vi "Master_NavigationLoop.vi"(8 "error in (no error)":errorcluster) -> (0 "error out":errorcluster)   [LabVIEW 2017]
uses:
  TypeDef_LoopPeriods.ctl
  DAQ/Master_DataControl.ctl
  DAQ/TypeDef_cRIOData.ctl
  IMU/TypeDef_IMUData.ctl
  CAN/TypeDef_BMSData.ctl
  CAN/TypeDef_BMS_Status.ctl
  CAN/MotorController/fixedMotorData.ctl
  CAN/MotorController/MotorStatus.ctl
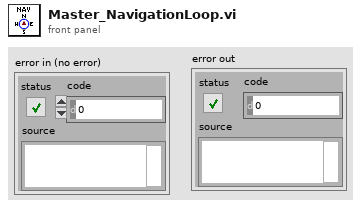
[diagram p1: front panel]
types:
  T1 = typedef "TypeDef_LoopPeriods.ctl" = cluster{"Control Period":i64, "DAQ Period":u32, "IMU Period":u32, "CAN Period":i64, "Nav Period":u32}
  T2 = typedef "Master_DataControl.ctl" = cluster{"cRIO Data":T3, "IMU Data":T4, "BMS Data":T5, "Motor Data":T7}
  T3 = typedef "TypeDef_cRIOData.ctl" = cluster{"Time (ms)":dbl, "24V Battery (V)":dbl, "LowV Current (A)":dbl, "Fiducial Sensor (V)":dbl, "PV Pressure (psig)":dbl, "Flow Sensor (V)":dbl, "Temp Fairing (F)":dbl, "Temp Reservoir (F)":dbl, "HallEffect Right (in)":dbl, "HallEffect Left (in)":dbl, "PT Tank (psig)":dbl, "PT Clamp Right (psig)":dbl, "PT Clamp Left (psig)":dbl, "PT Brake (psig)":dbl, "PT Cooling (psig)":dbl, "Displacement (ft)":dbl, "Velocity (ft/s)":dbl}
  T4 = typedef "TypeDef_IMUData.ctl" = cluster{"x acceleration (g)":dbl, "Pressure (psia)":dbl, "Temperature (F)":dbl}
  T5 = typedef "TypeDef_BMSData.ctl" = cluster{"Max Cell Voltage (V)":dbl, "Max Cell ID":dbl, "Min Cell Voltage (V)":dbl, "Min Cell ID":dbl, "State of Charge (%)":dbl, "Average Voltage (V)":dbl, "Voltage Delta (V)":dbl, "Pack Current (A)":dbl, "Pack Voltage (V)":dbl, "Max Resistance (Ohm)":dbl, "Min Resistance (Ohm)":dbl, "Average Resistance (Ohm)":dbl, "Delta Resistance (Ohm)":dbl, "Highest Temperature(F)":dbl, "BmsStatus":T6}
  T6 = typedef "TypeDef_BMS_Status.ctl" = cluster{"isFault":bool, "isolationMonitoring":bool}
  T7 = typedef "fixedMotorData.ctl" = cluster{"Velo (RPM)":dbl, "MotorTemp(F)":dbl, "CtrlTemp(F)":dbl, "DcLinkVolt(V)":dbl, "ErrorCode":dbl, "motorStatus":T8, "isAlive":bool, "motorControllerState":u16}
  T8 = typedef "MotorStatus.ctl" = cluster{"isReady":bool, "isOn":bool, "isOperEn":bool, "isFault":bool, "isVoltEn":bool, "targetReached":bool, "isWarning":bool}
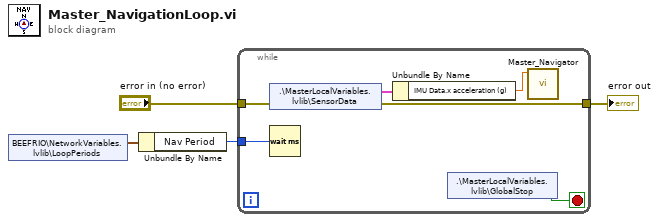
[diagram p0: block diagram]
diagram:
  n1 = shared-variable "BEEFRIO\\NetworkVariables.lvlib\\LoopPeriods"() -> (w3:T1)  [unwired: 1 in, 1 out]
  n2 = Unbundle By Name(w3) -> ("Nav Period"=w2:u32)
  n3 = while {
    tunnel: "error in (no error)" -> [w9]
    tunnel: w2 -> [w6]
    tunnel: [w5] -> w1
    stop <- w7 stop-if-true
    n4 = shared-variable ".\\MasterLocalVariables.lvlib\\SensorData"(error in=w9) -> (w10:T2, error out=w5:errorcluster)
    n5 = Wait (ms)(milliseconds to wait=w6) -> ()  [unwired: 1 out]
    n6 = Unbundle By Name(w10) -> ("IMU Data.x acceleration (g)"=w8:dbl)
    n7 = shared-variable ".\\MasterLocalVariables.lvlib\\GlobalStop"() -> (w7:bool)  [unwired: 1 in, 1 out]
    n8 = call "Master_Navigator.vi"("x acceleration (g)"=w8) -> ()  [unwired: 10 in, 1 out]
  }
  "error out" <- w1
